vi "BuildSpec Example.vi"() -> ()   [LabVIEW 2013]
uses:
  <vilib>/LabVIEW Open Source Project/Cron Scheduler/Job/Job Report -- cluster.ctl
  Job.BuildSpec/BuildSpec Job Configuration -- cluster.ctl
  Job.BuildSpec/Job.BuildSpec.lvclass
  <vilib>/LabVIEW Open Source Project/Cron Scheduler/Job/Job.lvclass/Job.ctl
  <vilib>/LabVIEW Open Source Project/Cron Scheduler/JobReport/JobReport.lvclass/JobReport.ctl
  <vilib>/LabVIEW Open Source Project/Cron Scheduler/Job/Job.lvclass
  <vilib>/LabVIEW Open Source Project/Cron Scheduler/Cron/Create Cron Expression.vi
  <vilib>/LabVIEW Open Source Project/Cron Scheduler/Cron/Compute Next Cron.vi
  <vilib>/LabVIEW Open Source Project/Cron Scheduler/Cron.Quartz/Cron.Quartz.lvclass
  <vilib>/LabVIEW Open Source Project/Cron Scheduler/openCron.lvlib
  <vilib>/LabVIEW Open Source Project/Cron Scheduler/JobReport/JobReport.lvclass
panel:
  out "exception message":string
  in  "BuildSpec Job Config":T1={"Project Path"=path "", "Build Name"="", "Target"="My Computer", "Clean"=FALSE, "Deploy"=FALSE}
  out "% Complete":dbl
  out "last error":errorcluster
  in  "Kill Job":bool
  in  "Abort Job":bool
  out "Job Report":T2
  out "Map":variant
  in  "Cron Expression":string="0 0 18 ? * *"
  out "syntax valid?":bool
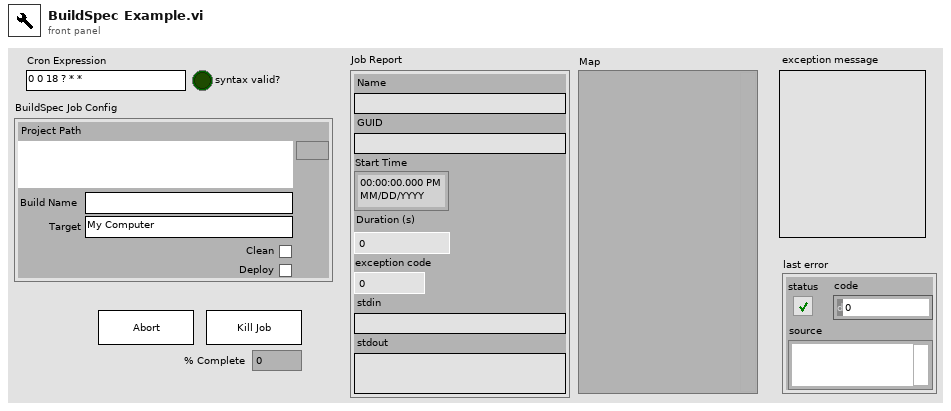
[diagram p1: front panel]
types:
  T1 = typedef "Job.BuildSpec.lvclass/BuildSpec Job Configuration -- cluster.ctl" = cluster{"Project Path":path, "Build Name":string, "Target":string, "Clean":bool, "Deploy":bool}
  T2 = typedef "openCronJob.lvlib/JobReport.lvclass/Job Report -- cluster.ctl" = cluster{"Name":string, "GUID":string, "Start Time":timestamp, "Duration (s)":dbl, "exception code":i32, "stdin":string, "stdout":string}
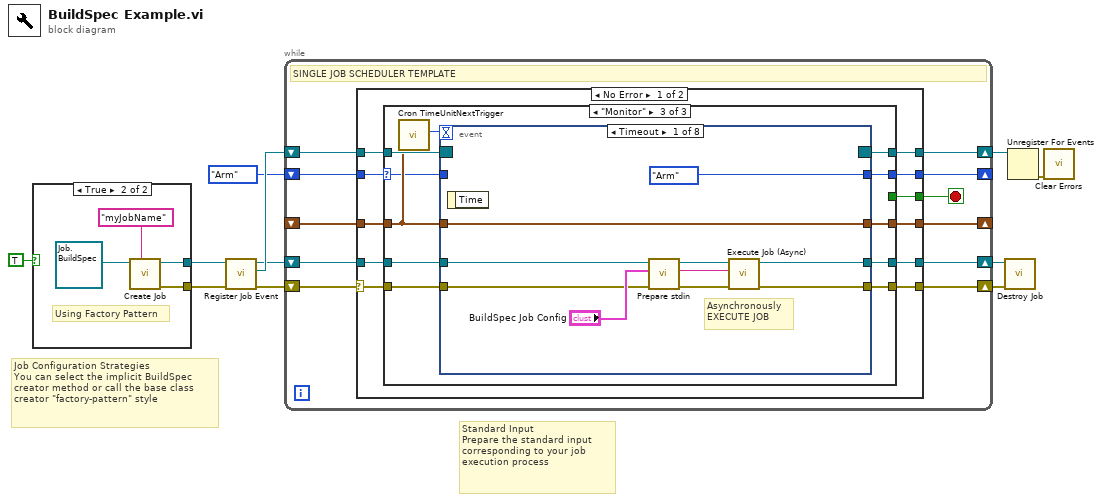
[diagram p0: block diagram]
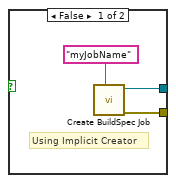
[diagram p2: hidden frame]
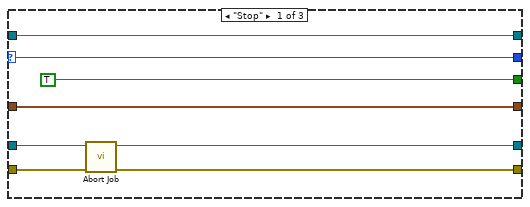
[diagram p3: hidden frame]
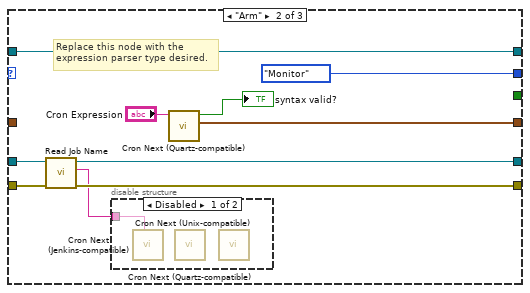
[diagram p4: hidden frame]
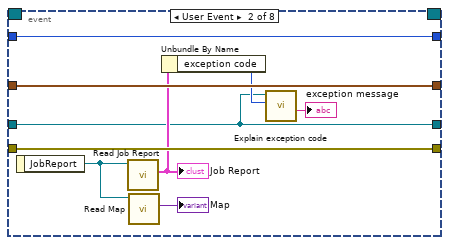
[diagram p6: hidden frame]
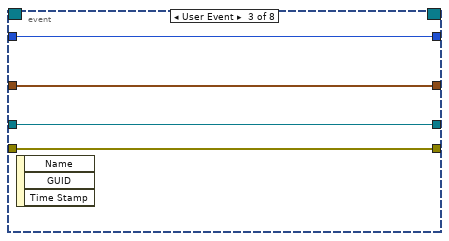
[diagram p7: hidden frame]
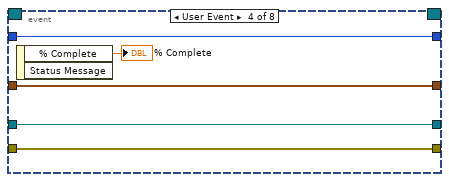
[diagram p8: hidden frame]
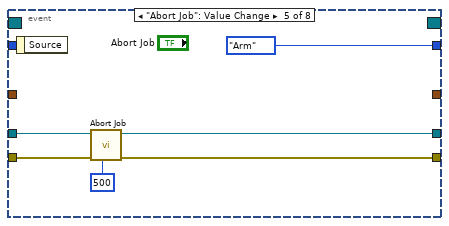
[diagram p9: hidden frame]
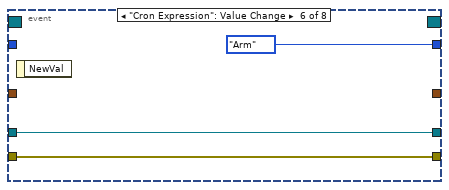
[diagram p10: hidden frame]
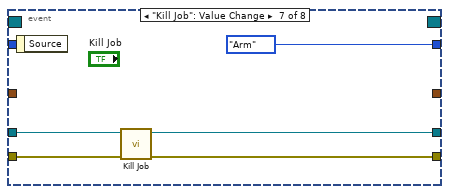
[diagram p11: hidden frame]
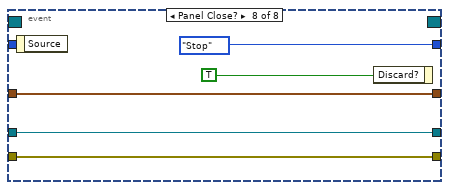
[diagram p12: hidden frame]
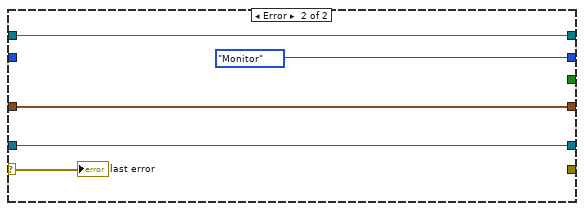
[diagram p13: hidden frame]
diagram:
  # "Job Configuration Strategies\nYou can select the implicit BuildSpec creator method or call the base class creator \"factory-pattern\" style"
  # "Standard Input\nPrepare the standard input corresponding to your job execution process"
  n1 = case shown="True" TRUE {
    tunnel: [w11 w17] -> w3
    tunnel: [w12 w16] -> w2
    frame False {
      # "Using Implicit Creator"
      n2 = call "Create BuildSpec Job.vi"("Job Name"="myJobName") -> ("error out"=w11:errorcluster, "Job.BuildSpec"=w12:refnum<class "Job.BuildSpec.lvclass">)  [unwired: 9 in]
    }
    frame True {
      # "Using Factory Pattern"
      n3 = call <vilib>:"Create Job.vi"("Job Name"="myJobName", "Job in"=refnum<class "Job.BuildSpec.lvclass"> refnum ("Job.BuildSpec")) -> ("error out"=w17:errorcluster, "Job"=w16:refnum<class "Job.BuildSpec.lvclass">)  [unwired: 8 in]
    }
  }
  n4 = call <vilib>:"Register Job Event.vi"("Job in"=w2) -> ("Job Event Registration"=w10:refnum<event-registration>, "Job out"=w8:refnum<class "Job.BuildSpec.lvclass">)  [unwired: 9 in]
  n5 = while {
    shift-right: [w27] -> _
    shift-left: _ -> [w28]
    shift-right: [w25] -> _
    shift-left: enum16{"Arm", "Stop", "Monitor"}."Arm" -> [w26]
    shift-right: [w22] -> w5
    shift-left: w10 -> [w23]
    shift-right: [w20] -> w7
    shift-left: w8 -> [w21]
    shift-right: [w19] -> w9
    shift-left: w3 -> [w18]
    stop <- w24 stop-if-true
    # "SINGLE JOB SCHEDULER TEMPLATE"
    n6 = case shown="No Error" w18 {
      selector: w18 -> [w29 w117]
      tunnel: w28 -> [w39 w119]
      tunnel: [w38 w119] -> w27
      tunnel: w26 -> [w37 _]
      tunnel: [w36 enum16{"Arm", "Stop", "Monitor"}."Monitor"] -> w25
      tunnel: [w35 _] -> w24
      tunnel: w23 -> [w34 w121]
      tunnel: [w33 w121] -> w22
      tunnel: w21 -> [w32 w118]
      tunnel: [w31 w118] -> w20
      tunnel: [w30 _] -> w19
      frame No Error {
        n7 = case shown="\"Monitor\"" w37 {
          selector: w37 -> [w47 _ w61]
          tunnel: w39 -> [w45 _ w64]
          tunnel: [w45 w56 w66] -> w38
          tunnel: [w47 enum16{"Arm", "Stop", "Monitor"}."Monitor" w67] -> w36
          tunnel: [TRUE _ _] -> w35
          tunnel: w34 -> [w44 w57 w69]
          tunnel: [w44 w57 w68] -> w33
          tunnel: w32 -> [w43 w50 w63]
          tunnel: [w42 w49 w62] -> w31
          tunnel: w29 -> [w41 w52 w60]
          tunnel: [w40 w51 w59] -> w30
          frame "Stop" {
            n8 = call <vilib>:"Abort Job.vi"("error in (no error)"=w41, "Job in"=w43) -> ("error out"=w40:errorcluster, "Job out"=w42:refnum<class "Job.BuildSpec.lvclass">)  [unwired: 5 in, 3 out]
          }
          frame "Arm" {
            # "Replace this node with the\nexpression parser type desired."
            n9 = call <vilib>:"Read Job Name.vi"("error in (no error)"=w52, "Job in"=w50) -> ("error out"=w51:errorcluster, "Name"=w48:string, "Job out"=w49:refnum<class "Job.BuildSpec.lvclass">)  [unwired: 7 in]
            n10 = disable-structure shown="Disabled" {
              disable-tunnel: w48 -> [w58 _]
              frame Disabled {
                n11 = call <vilib>:"Cron Next (Jenkins-compatible).vi"("Job Name"=w58) -> ()  [unwired: 8 in, 3 out]
                n12 = call <vilib>:"Cron Next (Quartz-compatible).vi"() -> ()  [unwired: 9 in, 3 out]
                n13 = call <vilib>:"Cron Next (Unix-compatible).vi"() -> ()  [unwired: 9 in, 3 out]
              }
              frame Enabled {
              }
            }
            n14 = call <vilib>:"Cron Next (Quartz-compatible).vi"("Cron Expression"="Cron Expression") -> ("Next Occurence"=w56:timestamp, "syntax valid?"=→"syntax valid?":bool)  [unwired: 8 in, 1 out]
          }
          frame "Monitor" {
            n15 = call <vilib>:"Cron TimeUnitNextTrigger.vi"("Next Occurence"=w64) -> ("next event (ms)"=w65:i32)  [unwired: 10 in]
            n16 = event shown="[0] Timeout" {
              selector: w69 -> [_ _ _ _ _ _ _ _]
              dyn-events: [_ _ _ _ _ _ _ _] -> w68
              timeout: w65 -> [_ _ _ _ _ _ _ _]
              tunnel: [enum16{"Arm", "Stop", "Monitor"}."Arm" w87 w91 w96 enum16{"Arm", "Stop", "Monitor"}."Arm" enum16{"Arm", "Stop", "Monitor"}."Arm" enum16{"Arm", "Stop", "Monitor"}."Arm" enum16{"Arm", "Stop", "Monitor"}."Stop"] -> w67
              tunnel: [w76 w88 w92 w97 _ _ _ w114] -> w66
              tunnel: w64 -> [w76 w88 w92 w97 _ _ _ w114]
              tunnel: w63 -> [w75 w80 w90 w95 w102 w105 w110 w113]
              tunnel: [w78 w80 w90 w95 w101 w105 w109 w113] -> w62
              tunnel: w61 -> [_ w87 w91 w96 _ _ _ _]
              tunnel: w60 -> [w71 w86 w89 w94 w99 w104 w108 w112]
              tunnel: [w77 w86 w89 w94 w98 w104 w107 w112] -> w59
              event Timeout {
                # "Asynchronously\nEXECUTE JOB"
                n17 = event-data() -> ()  [unwired: 1 in, 1 out]
                n18 = call "Prepare stdin.vi"("error in (no error)"=w71, "BuildSpec Job Config"="BuildSpec Job Config", "Job.BuildSpec in"=w75) -> ("error out"=w70:errorcluster, "Stdin"=w72:string, "Job.BuildSpec out"=w73:refnum<class "Job.BuildSpec.lvclass">)  [unwired: 6 in]
                n19 = call <vilib>:"Execute Job (Async).vi"("error in (no error)"=w70, "stdin"=w72, "Job in"=w73) -> ("error out"=w77:errorcluster, "Job out"=w78:refnum<class "Job.BuildSpec.lvclass">)  [unwired: 6 in, 1 out]
              }
              event User Event {
                n20 = event-data() -> ("JobReport"=w85:refnum<class "JobReport.lvclass">)  [unwired: 1 in]
                n21 = call <vilib>:"Read Job Report.vi"("JobReport in"=w85) -> ("Job Report"=w83:T2)  [unwired: 8 in, 2 out]
                "Job Report" <- w83
                n22 = call <vilib>:"Read Map.vi"("JobReport in"=w85) -> ("Map"=→"Map":variant)  [unwired: 8 in, 2 out]
                n23 = Unbundle By Name(w83) -> ("exception code"=w81:i32)
                n24 = call <vilib>:"Explain exception code.vi"("exception"=w81, "Job type"=w80) -> ("exception message"=→"exception message":string)  [unwired: 7 in, 2 out]
              }
              event User Event {
                n25 = event-data() -> ()  [unwired: 1 in, 3 out]
              }
              event User Event {
                n26 = event-data() -> ("% Complete"=→"% Complete":dbl)  [unwired: 1 in, 1 out]
              }
              event "Abort Job": Value Change {
                n27 = event-data() -> ()  [unwired: 1 in, 1 out]
                n28 = call <vilib>:"Abort Job.vi"("timeout (500 ms)"=500, "error in (no error)"=w99, "Job in"=w102) -> ("error out"=w98:errorcluster, "Job out"=w101:refnum<class "Job.BuildSpec.lvclass">)  [unwired: 4 in, 3 out]
              }
              event "Cron Expression": Value Change {
                n29 = event-data() -> ()  [unwired: 1 in, 1 out]
              }
              event "Kill Job": Value Change {
                n30 = event-data() -> ()  [unwired: 1 in, 1 out]
                n31 = call <vilib>:"Kill Job.vi"("error in (no error)"=w108, "Job in"=w110) -> ("error out"=w107:errorcluster, "Job out"=w109:refnum<class "Job.BuildSpec.lvclass">)  [unwired: 8 in]
              }
              event Panel Close? {
                n32 = event-data() -> ()  [unwired: 1 in, 1 out]
                n33 = event-data("Discard?"=TRUE) -> ()  [unwired: 1 in, 1 out]
              }
            }
          }
        }
      }
      frame Error {
        "last error" <- w117
      }
    }
  }
  n34 = call <vilib>:"Destroy Job.vi"("error in (no error)"=w9, "Job in"=w7) -> ()  [unwired: 8 in, 2 out]
  n35 = Unregister For Events(event registration refnum=w5) -> (error out=w6:errorcluster)  [unwired: 1 in]
  n36 = call <vilib>:"Clear Errors.vi"("error in (no error)"=w6) -> ()  [unwired: 6 in, 1 out]
